vi "Construct Base.vi"(0 "Execution Unit Implementation (default object)":refnum<class "Execution Unit.lvclass">, 1 "identifier":string, 2 "Channel":u8, 3 "error in (no error)":errorcluster, 4 "async loop rate hz":dbl) -> (7 "Execution Unit Out":refnum<class "Execution Unit.lvclass">, 10 "error out":errorcluster)   [LabVIEW 2020, in "AIM ARINC 664 Engine.lvlib" / "Implementation.lvlib" / "Execution Unit.lvclass"]
uses:
  Execution Unit.lvclass
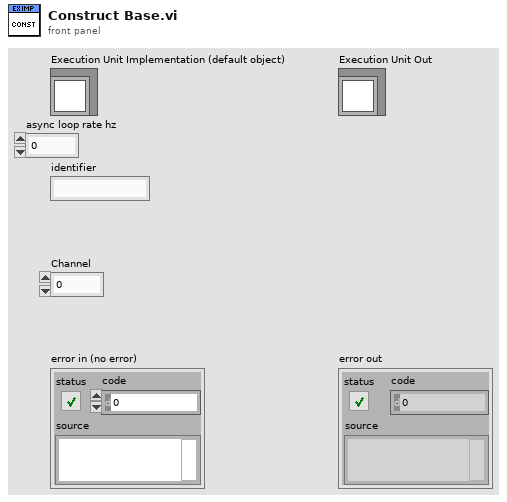
[diagram p1: front panel]
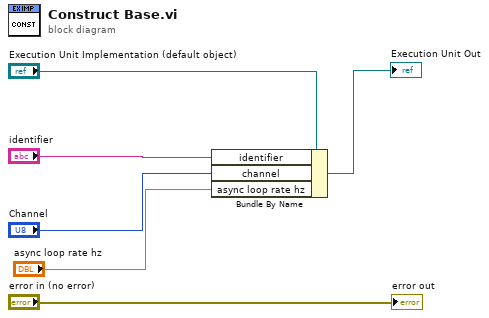
[diagram p0: block diagram]
diagram:
  n1 = Bundle By Name(cluster="Execution Unit Implementation (default object)", "identifier"="identifier", "channel"="Channel", "async loop rate hz"="async loop rate hz") -> (→"Execution Unit Out":refnum<class "Execution Unit.lvclass">)
  "error out" <- "error in (no error)"
